vi "bode plot.vi"() -> ()   [LabVIEW 2020]
uses:
  <vilib>/addons/Control Design/_Model Construction/Data Typedefs.llb/CD Bode Data.ctl
  <vilib>/addons/Control Design/_Model Construction/Data Typedefs.llb/CD Plot Types Enum.ctl
  <vilib>/addons/Control Design/_Model Construction/Model Creation.llb/Model Creation SubVI/cd_Create Transfer Function Model.vi
  <vilib>/addons/Control Design/_Frequency Response Analysis/Frequency Response.llb/Frequency Response subVI/cd_Bode (Transfer Function).vi
  <vilib>/addons/Control Design/_Utility/Model Viewer.llb/Model Viewer SubVI/cd_Draw Transfer Function Equation (TF).vi
  <vilib>/addons/Control Design/_Utility/NI_CD_Model Viewer.lvlib
  <vilib>/addons/Control Design/_Model Construction/NI_LinSys_Model Creation.lvlib
  <vilib>/addons/Control Design/_Frequency Response Analysis/NI_CD_Frequency Response.lvlib
  <vilib>/addons/Control Design/_Model Construction/NI_LinSys_Data Typedefs.lvlib
panel:
  out "Bode Data":T1={"Frequency"=[], "Magnitude"=[], "Phase"=[], "plot type"=enum."bode-phase"} {"Phase" format="%#.6g"; "Magnitude" format="%#.6g"; "Frequency" format="%#.6g"}
  out "Bode Phase":cluster{"W":dbl[], "Magnitude":dbl[]}[](graph)
  out "Bode Magnitude":cluster{"W":dbl[], "Magnitude":dbl[]}[](graph)
  in  "Delay":dbl=nan format="%.2f"
  in  "Denominator":dbl[](array[numeric]) format="%#.5g"
  in  "Numerator":dbl[](array[numeric]) format="%#.5g"
  out "Equation":picture
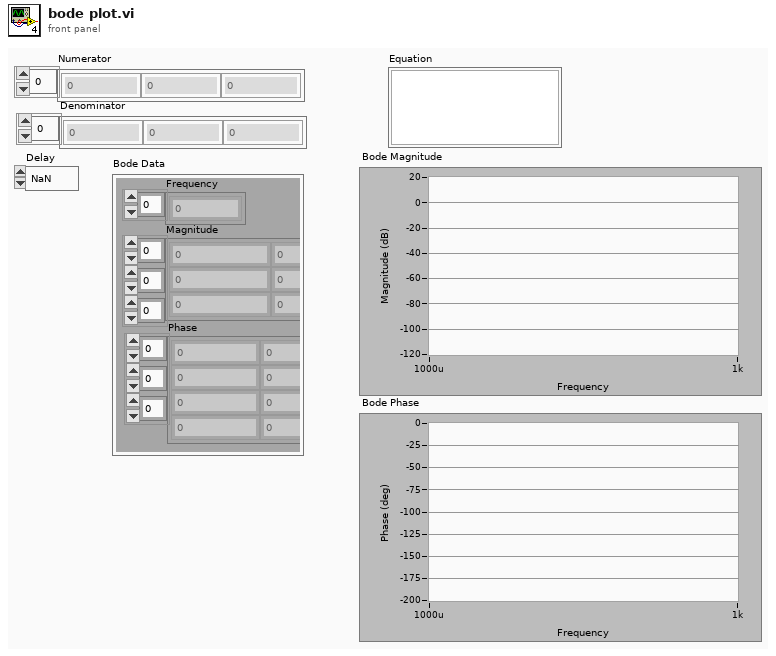
[diagram p1: front panel]
types:
  T1 = typedef "NI_LinSys_Data Typedefs.lvlib/CD Bode Data.ctl" = cluster{"Frequency":dbl[], "Magnitude":dbl[][][], "Phase":dbl[][][], "plot type":T2}
  T2 = typedef "NI_LinSys_Data Typedefs.lvlib/CD Plot Types Enum.ctl" = enum16{"bode-magnitude", "bode-phase", "nichols", "nyquist", "singular values", "step", "impulse", "initial", "simulation", "nyquist with separation"}
  T3 = typedef "NI_LinSys_Model Typedefs.lvlib/CD Transfer Function Model (MIMO).ctl" = cluster{"properties":T4, "transfer function(s)":T5[][]}
  T4 = typedef "NI_LinSys_Model Typedefs.lvlib/CD General Elements.ctl" = cluster{"Model name":string, "Input names":string[], "Output names":string[], "Input Delays":dbl[], "Output Delays":dbl[], "Sampling Time":dbl, "Notes":string}
  T5 = typedef "NI_LinSys_Model Typedefs.lvlib/CD Transfer Function Model (SISO).ctl" = cluster{"Numerator":dbl[], "Denominator":dbl[], "delay":dbl}
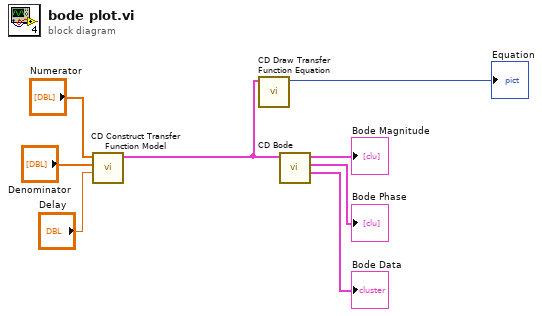
[diagram p0: block diagram]
diagram:
  n1 = call-poly <vilib>:"CD Construct Transfer Function Model.vi"("Delay"="Delay", "Denominator"="Denominator", "Numerator"="Numerator") -> ("Transfer Function Model"=w3:T3)  [unwired: 7 in, 1 out]
  n2 = call-poly <vilib>:"CD Draw Transfer Function Equation.vi"("Transfer Function Model"=w3) -> ("Equation"=→"Equation":picture)  [unwired: 8 in, 2 out]
  n3 = call-poly <vilib>:"CD Bode.vi"("Transfer Function Model"=w3) -> ("Bode Data"=→"Bode Data":T1, "Bode Phase"=→"Bode Phase":cluster{"W":dbl[], "Magnitude":dbl[]}[], "Bode Magnitude"=→"Bode Magnitude":cluster{"W":dbl[], "Magnitude":dbl[]}[])  [unwired: 6 in, 2 out]
